vi "AVS_GetAnalogIn.vi"(0 "a_hDevice":i32, 7 "a_AnalogInId":u8, 11 "a_pAnalogIn":sgl) -> (4 "Output Value":i32, 15 "a_pAnalogIn":sgl)   [LabVIEW 2018]
uses:
  avaspecx64.dll
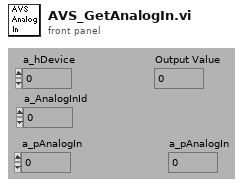
[diagram p1: front panel]
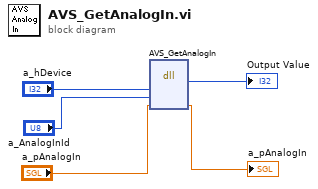
[diagram p0: block diagram]
diagram:
  n1 = dll-call lib="C:/AvaSpecX64-DLL_9.7/examples/LabView/LabViewSingleChan/avaspecx64.dll" fn="AVS_GetAnalogIn"("a_hDevice"="a_hDevice", "a_AnalogInId"="a_AnalogInId", "a_pAnalogIn"="a_pAnalogIn") -> ("return type"=→"Output Value":i32, "a_pAnalogIn"=→"a_pAnalogIn":sgl)  [unwired: 5 in, 2 out]
